vi "toml_parse_number.vi"(8 "error in (no error)":errorcluster, 11 "string":string) -> (0 "error out":errorcluster, 2 "value":variant, 3 "remaining string":string)   [LabVIEW 2017]
uses:
  <vilib>/Utility/error.llb/Error Cluster From Error Code.vi
  <vilib>/regexp/Match Regular Expression.xnode
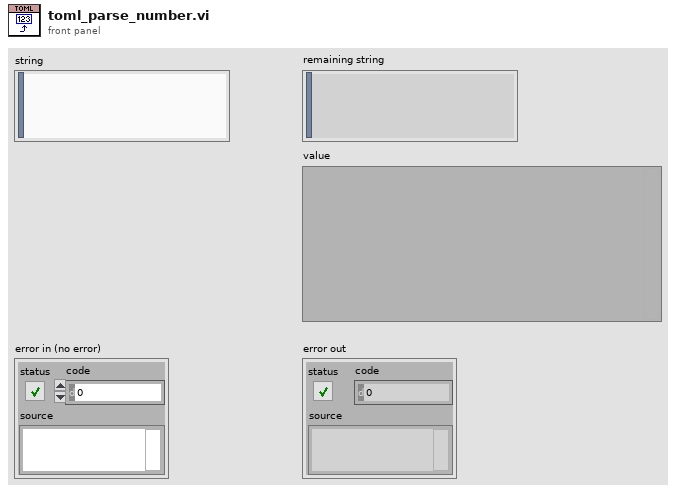
[diagram p1: front panel]
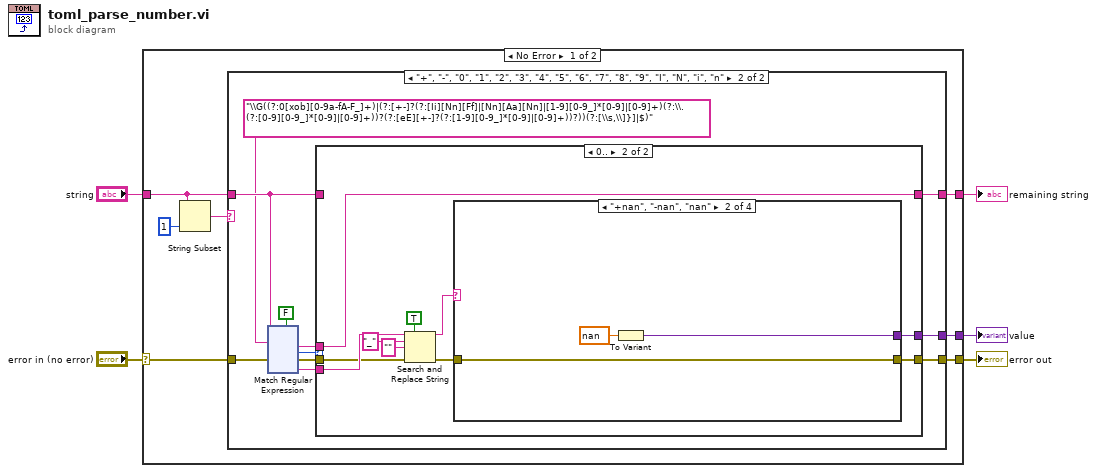
[diagram p0: block diagram]
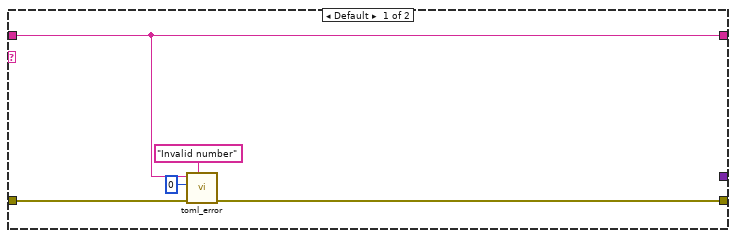
[diagram p2: hidden frame]
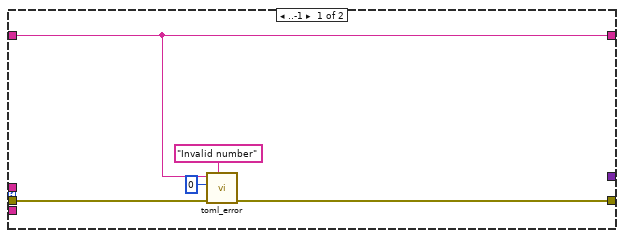
[diagram p3: hidden frame]
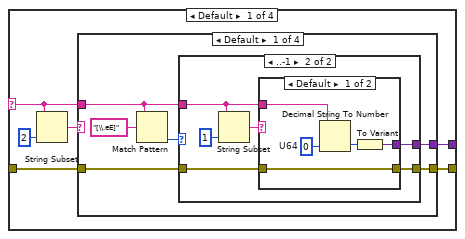
[diagram p4: hidden frame]
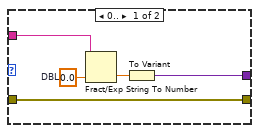
[diagram p5: hidden frame]
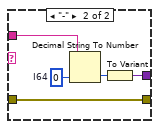
[diagram p6: hidden frame]
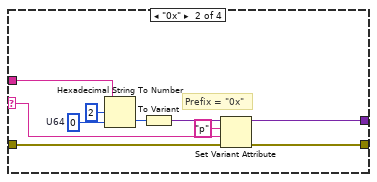
[diagram p7: hidden frame]
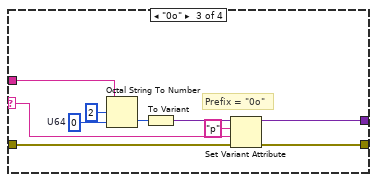
[diagram p8: hidden frame]
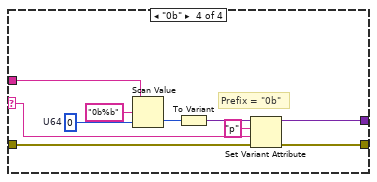
[diagram p9: hidden frame]
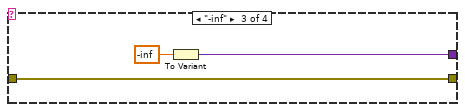
[diagram p10: hidden frame]
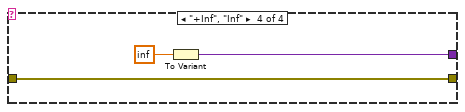
[diagram p11: hidden frame]
diagram:
  n1 = case shown="No Error" "error in (no error)" {
    selector: "error in (no error)" -> [w12 w233]
    tunnel: "string" -> [w11 w232]
    tunnel: [w9 w233] -> w3
    tunnel: [w7 w232] -> w2
    tunnel: [w6 _] -> w1
    frame No Error {
      n2 = String Subset(string=w11, length (rest)=1 ("length (rest)")) -> (substring=w8:string)  [unwired: 1 in]
      n3 = case shown="\"+\", \"-\", \"0\", \"1\", \"2\", \"3\", \"4\", \"5\", \"6\", \"7\", \"8\", \"9\", \"I\", \"N\", \"i\", \"n\"" w8 {
        tunnel: w12 -> [w17 w27]
        tunnel: w11 -> [w15 w21]
        tunnel: [w16 w24] -> w9
        tunnel: [w15 w22] -> w7
        tunnel: [_ w19] -> w6
        frame Default {
          n4 = call "toml_error.vi"("message"="Invalid number" ("source"), "error in (no error)"=w17, "offset (0)"=0, "toml"=w15) -> ("error out"=w16:errorcluster)  [unwired: 7 in]
        }
        frame "+", "-", "0", "1", "2", "3", "4", "5", "6", "7", "8", "9", "I", "N", "i", "n" {
          n5 = xnode "Match Regular Expression"("input string"=w21, "regular expression"="\\G((?:0[xob][0-9a-fA-F_]+)|(?:[+-]?(?:[Ii][Nn][Ff]|[Nn][Aa][Nn]|[1-9][0-9_]*[0-9]|[0-9]+)(?:\\.(?:[0-9][0-9_]*[0-9]|[0-9]+))?(?:[eE][+-]?(?:[1-9][0-9_]*[0-9]|[0-9]+))?))(?:[\\s,\\]}]|$)", "error in"=w27, "multiline? (F)"=FALSE) -> ("after match"=w20:string, "offset past match"=w25:i32, "error out"=w23:errorcluster, "submatch 1"=w26:string)  [unwired: 2 in, 2 out]
          n6 = case shown="0.." w25 {
            tunnel: w26 -> [_ w41]
            tunnel: [w30 w42] -> w24
            tunnel: w23 -> [w31 w37]
            tunnel: [w29 w43] -> w22
            tunnel: w21 -> [w29 _]
            tunnel: w20 -> [_ w43]
            tunnel: [_ w34] -> w19
            frame ..-1 {
              n7 = call "toml_error.vi"("message"="Invalid number" ("source"), "error in (no error)"=w31, "offset (0)"=0, "toml"=w29) -> ("error out"=w30:errorcluster)  [unwired: 7 in]
            }
            frame 0.. {
              n8 = Search and Replace String(replace all?=TRUE ("replace all? (F)"), input string=w41, search string="_", replace string="" ("replace string (\"\")"), error in=w37) -> (result string=w40:string, error out=w36:errorcluster)  [unwired: 3 in, 2 out]
              n9 = case shown="\"+nan\", \"-nan\", \"nan\"" w40 {
                selector: w40 -> [w47 _ _ _]
                tunnel: [w49 w109 w112 w115] -> w42
                tunnel: w36 -> [w48 w109 w112 w115]
                tunnel: [w46 w107 w110 w113] -> w34
                frame Default {
                  n10 = String Subset(string=w47, length (rest)=2 ("length (rest)")) -> (substring=w44:string)  [unwired: 1 in]
                  n11 = case shown="Default" w44 {
                    selector: w44 -> [_ w77 w87 w97]
                    tunnel: [w55 w81 w90 w100] -> w49
                    tunnel: w48 -> [w54 w82 w91 w101]
                    tunnel: [w53 w79 w88 w98] -> w46
                    tunnel: w47 -> [w51 w84 w94 w103]
                    frame Default {
                      n12 = Match Pattern(string=w51, regular expression="[\\.eE]") -> (offset past match=w50:i32)  [unwired: 1 in, 3 out]
                      n13 = case shown="..-1" w50 {
                        tunnel: w51 -> [w60 w64]
                        tunnel: [w56 w63] -> w55
                        tunnel: w54 -> [w56 w62]
                        tunnel: [w57 w61] -> w53
                        frame 0.. {
                          w59 = 0.0  # DBL
                          n14 = Fract/Exp String To Number(string=w60, default (0 dbl)=w59) -> (number=w58:dbl)  [unwired: 2 in, 1 out]
                          n15 = To Variant(anything=w58) -> (Variant=w57:variant)
                        }
                        frame ..-1 {
                          n16 = String Subset(string=w64, length (rest)=1 ("length (rest)")) -> (substring=w65:string)  [unwired: 1 in]
                          n17 = case shown="Default" w65 {
                            tunnel: w64 -> [w71 w76]
                            tunnel: [w68 w73] -> w63
                            tunnel: w62 -> [w68 w73]
                            tunnel: [w67 w72] -> w61
                            frame Default {
                              w69 = u64 0  # U64
                              n18 = Decimal String To Number(string=w71, default (0L)=w69) -> (number=w70:u64)  [unwired: 1 in, 1 out]
                              n19 = To Variant(anything=w70) -> (Variant=w67:variant)
                            }
                            frame "-" {
                              w74 = i64 0  # I64
                              n20 = Decimal String To Number(string=w76, default (0L)=w74) -> (number=w75:i64)  [unwired: 1 in, 1 out]
                              n21 = To Variant(anything=w75) -> (Variant=w72:variant)
                            }
                          }
                        }
                      }
                    }
                    frame "0x" {
                      w86 = u64 0  # U64
                      # "Prefix = \"0x\""
                      n22 = Hexadecimal String To Number(string=w84, offset=2, default (0uL)=w86) -> (number=w85:u64)  [unwired: 1 out]
                      n23 = To Variant(anything=w85) -> (Variant=w80:variant)
                      n24 = Set Variant Attribute(Variant=w80, name="p", value=w77, error in=w82) -> (Variant out=w79:variant, error out=w81:errorcluster)  [unwired: 1 out]
                    }
                    frame "0o" {
                      w96 = u64 0  # U64
                      # "Prefix = \"0o\""
                      n25 = Octal String To Number(2:w96, 3:2 ("offset"), 4:w94) -> (0:w95:u64)  [unwired: 1 out]
                      n26 = To Variant(anything=w95) -> (Variant=w89:variant)
                      n27 = Set Variant Attribute(Variant=w89, name="p", value=w87, error in=w91) -> (Variant out=w88:variant, error out=w90:errorcluster)  [unwired: 1 out]
                    }
                    frame "0b" {
                      w106 = u64 0  # U64
                      # "Prefix = \"0b\""
                      n28 = Scan Value(string=w103, format string="0b%b", default (0 dbl)=w106) -> (value=w104:u64)  [unwired: 1 out]
                      n29 = To Variant(anything=w104) -> (Variant=w99:variant)
                      n30 = Set Variant Attribute(Variant=w99, name="p", value=w97, error in=w101) -> (Variant out=w98:variant, error out=w100:errorcluster)  [unwired: 1 out]
                    }
                  }
                }
                frame "+nan", "-nan", "nan" {
                  n31 = To Variant(anything=nan) -> (Variant=w107:variant)
                }
                frame "-inf" {
                  n32 = To Variant(anything=-inf) -> (Variant=w110:variant)
                }
                frame "+Inf", "Inf" {
                  n33 = To Variant(anything=inf) -> (Variant=w113:variant)
                }
              }
            }
          }
        }
      }
    }
    frame Error {
    }
  }
  "error out" <- w3
  "remaining string" <- w2
  "value" <- w1
